vi "GE 5565PIORC.Registers.LISR.Local Memory Parity Error.Set.vi"(8 "error in (no error)":errorcluster, 10 "Local Memory Parity Error":bool, 11 "GE 5565PIORC in":refnum<class "GE 5565PIORC.lvclass">) -> (0 "error out":errorcluster, 3 "GE 5565PIORC out":refnum<class "GE 5565PIORC.lvclass">)   [LabVIEW 2016, in "GE 5565PIORC.lvclass"]
doc: "When this bit is high (1), one or more parity errors have been detected on local memory accesses. This bit is latched. Once set, it must be cleared by writing a zero to this bit location. Note that Bit 27 of the LCSR1 must be set high before parity is active. Also note that parity works only on 32-bit and 64-bit accesses. Word (16-bit) and byte (8-bit) memory write accesses are inhibited."
uses:
  GE 5565PIORC.lvclass
  GE 5565PIORC.Registers.RFM Control and Status.ctl
  GE 5565PIORC.Register.RFM Control and Status.Read (U32).vi
  Bit Manipulation.Set Bit (U32).vi
  GE 5565PIORC.Register.RFM Control and Status.Write (U32).vi
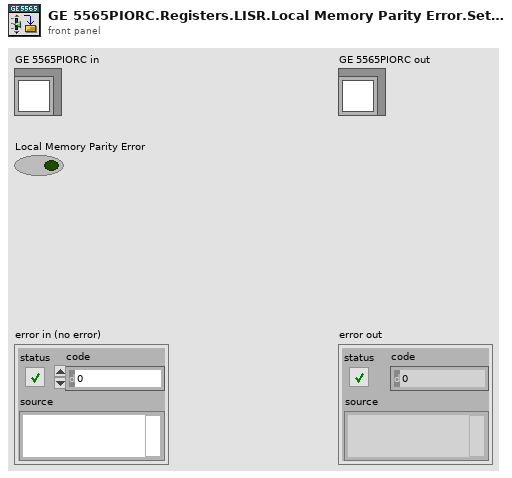
[diagram p1: front panel]
types:
  T1 = typedef "GE 5565PIORC.lvclass/GE 5565PIORC.Registers.RFM Control and Status.ctl" = u32
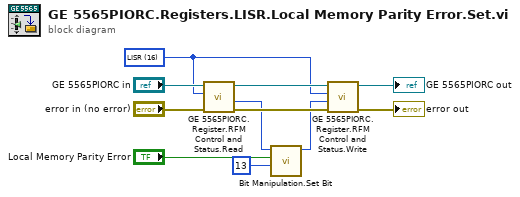
[diagram p0: block diagram]
diagram:
  w5 = T1 16 items=["BRV"=0, "BID"=1, "BRB"=2, "NID"=4, "LCSR1"=8, "LISR"=16, "LIER"=20, "NTD"=24, "NTN"=28, "NIC"=29, "ISD1"=32, "SID1"=36, "ISD2"=40, "SID2"=44, "ISD3"=48, "SID3"=52, "ISD4"=56, "SID4"=60] ("Register")
  n1 = call-poly "GE 5565PIORC.Register.RFM Control and Status.Read.vi"("error in (no error)"="error in (no error)", "Register"=w5, "GE 5565PIORC in"="GE 5565PIORC in") -> ("error out"=w11:errorcluster, "Value"=w3:u32, "GE 5565PIORC out"=w8:refnum<class "GE 5565PIORC.lvclass">)  [unwired: 6 in]
  n2 = call-poly "Bit Manipulation.Set Bit.vi"("bit index"=13, "bit"="Local Memory Parity Error", "packed value in"=w3) -> ("packed value out"=w2:u32)  [unwired: 8 in]
  n3 = call-poly "GE 5565PIORC.Register.RFM Control and Status.Write.vi"("error in (no error)"=w11, "Value"=w2, "Register"=w5, "GE 5565PIORC in"=w8) -> ("error out"=→"error out":errorcluster, "GE 5565PIORC out"=→"GE 5565PIORC out":refnum<class "GE 5565PIORC.lvclass">)  [unwired: 6 in]
